vi "zad8.vi"() -> ()   [LabVIEW 2025]
panel:
  out "XY Graph":cluster{dbl[], dbl[]}(graph)
  in  "MAX":i32
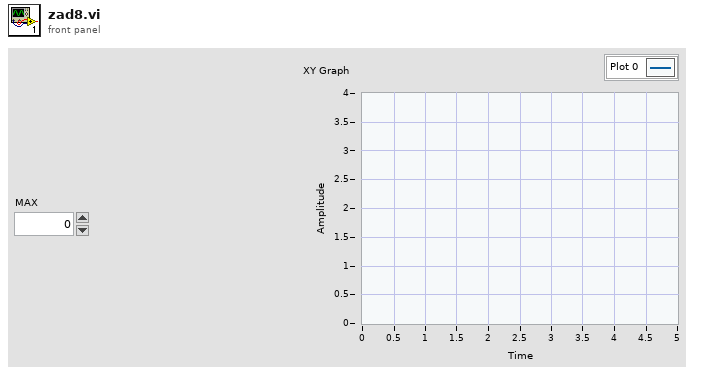
[diagram p1: front panel]
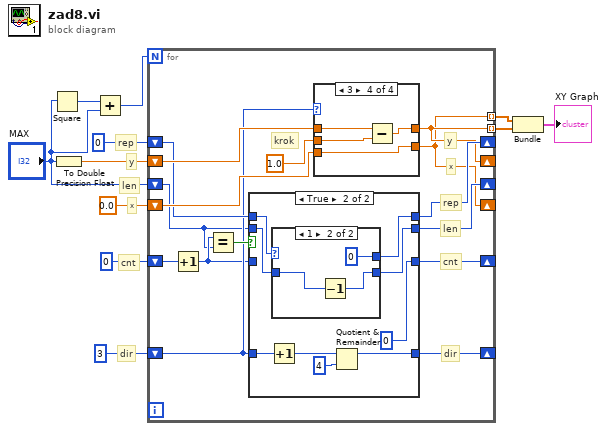
[diagram p0: block diagram]
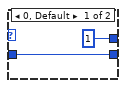
[diagram p3: hidden frame]
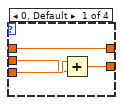
[diagram p4: hidden frame]
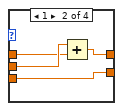
[diagram p5: hidden frame]
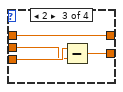
[diagram p6: hidden frame]
diagram:
  # "rep"
  # "len"
  # "cnt"
  # "x"
  # "y"
  # "dir"
  n1 = Square(x="MAX") -> (x^2=w3:i32)
  n2 = To Double Precision Float(number="MAX") -> (double precision float=w2:dbl)
  n3 = Add(x=w3, y="MAX") -> (x+y=w4:i32)
  n4 = for {
    N: w4 -> [_]
    shift-right: [w21] -> _
    shift-left: 3 -> [w19]
    shift-right: [w13] -> _
    shift-left: 0.0 -> [w26]
    shift-right: [w14] -> _
    shift-left: w2 -> [w25]
    shift-right: [w22] -> _
    shift-left: 0 -> [w16]
    shift-right: [w18] -> _
    shift-left: "MAX" -> [w12]
    shift-right: [w17] -> _
    shift-left: 0 -> [w20]
    tunnel: [w14] -> w5 mode=indexing
    tunnel: [w13] -> w6 mode=indexing
    # "x"
    # "y"
    # "rep"
    # "len"
    # "dir"
    # "cnt"
    # "krok"
    n5 = Increment(x=w16) -> (x+1=w15:i32)
    n6 = Equal?(x=w15, y=w12) -> (x = y?=w23:bool)
    n7 = case shown="True" w23 {
      tunnel: [w27 0] -> w22
      tunnel: [w28 w31] -> w21
      tunnel: w19 -> [w28 w37]
      tunnel: w20 -> [w29 w35]
      tunnel: w12 -> [w30 w34]
      tunnel: [w30 w33] -> w18
      tunnel: [w29 w32] -> w17
      tunnel: w15 -> [w27 _]
      frame False {
      }
      frame True {
        n8 = Increment(x=w37) -> (x+1=w36:i32)
        n9 = case shown="1" w35 {
          tunnel: w34 -> [w41 w43]
          tunnel: [w41 w42] -> w33
          tunnel: [1 0] -> w32
          frame 0, Default {
          }
          frame 1 {
            n10 = Decrement(x=w43) -> (x-1=w42:i32)
          }
        }
        n11 = Quotient & Remainder(x=w36, y=4) -> (x-y*floor(x/y)=w31:i32)  [unwired: 1 out]
      }
    }
    n12 = case shown="3" w19 {
      tunnel: w26 -> [w46 w52 w56 w58]
      tunnel: w25 -> [w48 w50 w54 w60]
      tunnel: [w48 w49 w54 w57] -> w14
      tunnel: [w47 w52 w53 w58] -> w13
      tunnel: 1.0 -> [w45 w51 w55 w59]
      frame 0, Default {
        n13 = Add(x=w46, y=w45) -> (x+y=w47:dbl)
      }
      frame 1 {
        n14 = Add(x=w51, y=w50) -> (x+y=w49:dbl)
      }
      frame 2 {
        n15 = Subtract(x=w56, y=w55) -> (x-y=w53:dbl)
      }
      frame 3 {
        n16 = Subtract(x=w60, y=w59) -> (x-y=w57:dbl)
      }
    }
  }
  n17 = Bundle(w6, w5) -> (→"XY Graph":cluster{dbl[], dbl[]})  [unwired: 1 in]
